vi "AddTexture.vi"(3 "error in (no error)":errorcluster, 4 "path to JPEG file":path=path "earth.jpg", 5 "object In":refnum<vi>) -> (0 "error out":errorcluster, 2 "object out":refnum<vi>)   [LabVIEW 2024]
uses:
  <vilib>/picture/3D Picture Control/NI_3D Picture Control.lvlib
panel:
  in  "Apply Mode":T1(ring)
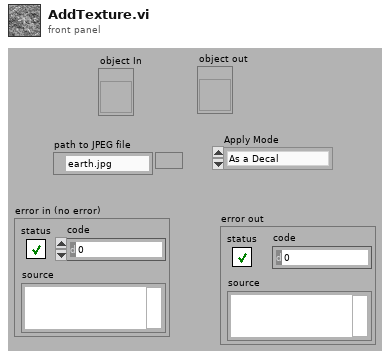
[diagram p1: front panel]
types:
  T1 = enum16{"As a Decal", "With Modulation", "With Blending", "As a replacement"}
  T2 = typedef "imagedata.ctl" = cluster{"image type":i32, "image depth":i32, "image":u8[], "mask":u8[], "colors":u32[], "Rectangle":cluster{"left":i16, "top":i16, "right":i16, "bottom":i16}}
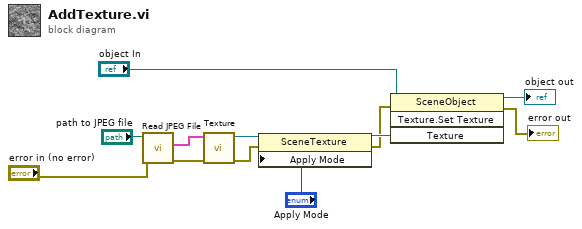
[diagram p0: block diagram]
diagram:
  n1 = call <vilib>:"Read JPEG File.vi"("error in (no error)"="error in (no error)", "path to JPEG file"="path to JPEG file") -> ("error out"=w8:errorcluster, "image data"=w11:T2)  [unwired: 8 out]
  n2 = call <vilib>:"Texture.vi"("error in (no error)"=w8, "Image"=w11) -> ("error out"=w2:errorcluster, "New Texture Refnum"=w5:refnum<vi>)  [unwired: 8 out]
  n3 = property class="SceneTexture"(reference=w5, error in=w2, "Apply Mode"="Apply Mode") -> (reference out=w3:refnum<vi>, error out=w1:errorcluster)
  n4 = invoke class="SceneObject" method="Texture.Set Texture"(reference="object In", error in=w1, "Texture"=w3) -> (reference out=→"object out":refnum<vi>, error out=→"error out":errorcluster)  [unwired: 1 in, 2 out]
